vi "generate_double_circ_trajectory.vi"(0 "TrajectoryTS090820Circular2D in":refnum<class "TrajectoryTS090820Circular2D.lvclass">, 1 "trajectory params":T1, 5 "error in (no error)":errorcluster) -> (14 "TrajectoryTS090820Circular2D out":refnum<class "TrajectoryTS090820Circular2D.lvclass">, 15 "trajectory":cluster{dbl[], dbl[], dbl[], dbl[]}, 19 "error out":errorcluster)   [LabVIEW 2010, in "TrajectoryTS090820Circular2D.lvclass"]
uses:
  TrajectoryTS090820Circular2D.lvclass
panel:
  out "dumping amplitude":dbl[](graph)
  out "points BEFORE equal-distribution":cluster{dbl, dbl}[](graph)
  out "intensity":dbl[](array[numeric])
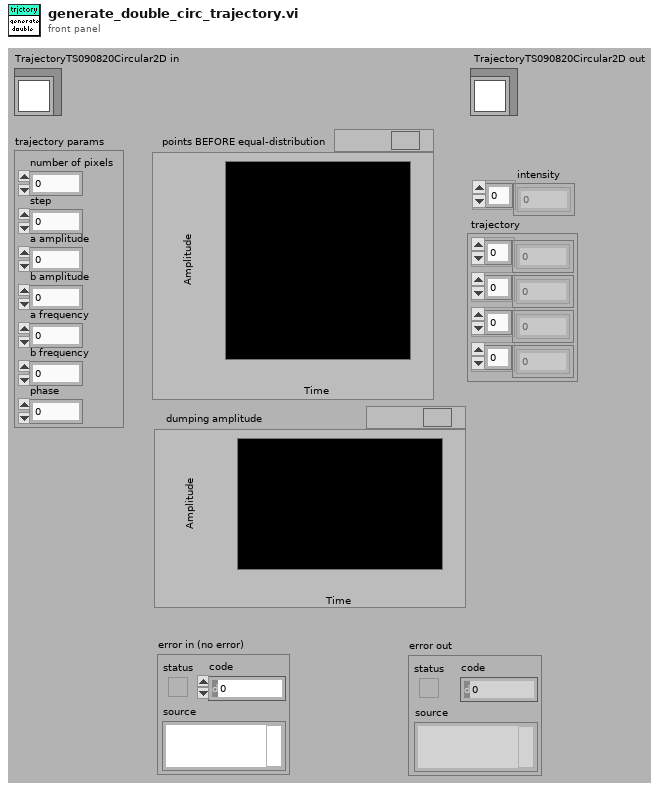
[diagram p1: front panel]
types:
  T1 = cluster{"number of pixels":i32, "step":dbl, "a amplitude":dbl, "b amplitude":dbl, "a frequency":dbl, "b frequency":dbl, "phase":dbl}
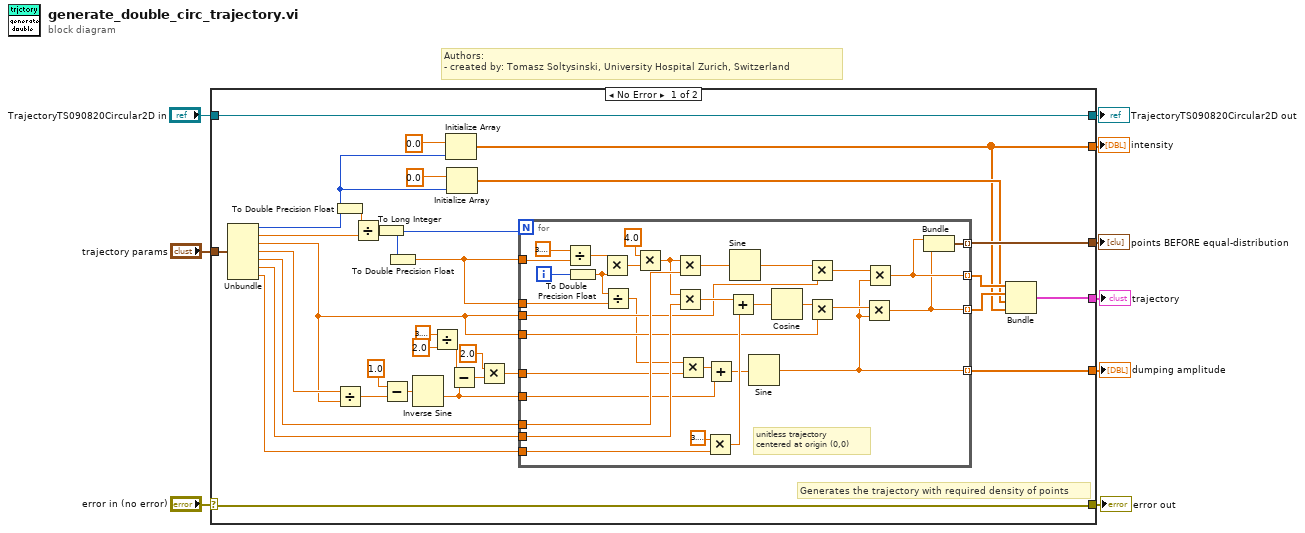
[diagram p0: block diagram]
diagram:
  # "Authors: \n- created by: Tomasz Soltysinski, University Hospital Zurich, Switzerland"
  n1 = case shown="No Error" "error in (no error)" {
    selector: "error in (no error)" -> [w42 w76]
    tunnel: [w42 w76] -> w9
    tunnel: [w24 w75] -> w7
    tunnel: "TrajectoryTS090820Circular2D in" -> [w24 w75]
    tunnel: [w27 _] -> w6
    tunnel: "trajectory params" -> [w37 _]
    tunnel: [w31 _] -> w4
    tunnel: [w26 _] -> w3
    tunnel: [w11 _] -> w1
    frame No Error {
      # "Generates the trajectory with required density of points"
      n2 = Unbundle(w37) -> ("number of pixels"=w36:i32, "step"=w35:dbl, "a amplitude"=w12:dbl, "b amplitude"=w13:dbl, "a frequency"=w34:dbl, "b frequency"=w33:dbl, "phase"=w32:dbl)
      n3 = To Double Precision Float(number=w36) -> (double precision float=w39:dbl)
      n4 = Divide(x=w13, y=w12) -> (x/y=w14:dbl)
      n5 = Divide(x=w39, y=w35) -> (x/y=w38:dbl)
      n6 = To Long Integer(number=w38) -> (32bit integer=w25:i32)
      n7 = Subtract(x=1.0, y=w14) -> (x-y=w22:dbl)
      n8 = To Double Precision Float(number=w25) -> (double precision float=w10:dbl)
      n9 = Inverse Sine(1:w22) -> (0:w15:dbl)
      n10 = Divide(x=3.141592653589793, y=2.0) -> (x/y=w19:dbl)
      n11 = Initialize Array(0.0 ("dimension size"), w36) -> (w27:dbl[])
      n12 = Initialize Array(0.0 ("dimension size"), w36) -> (w28:dbl[])
      n13 = Subtract(x=w19, y=w15) -> (x-y=w18:dbl)
      n14 = Multiply(x=2.0, y=w18) -> (x*y=w16:dbl)
      n15 = for {
        N: w25 -> [_]
        tunnel: w32 -> [w68]
        tunnel: w10 -> [w71]
        tunnel: w34 -> [w67]
        tunnel: w33 -> [w66]
        tunnel: [w49] -> w30 mode=indexing
        tunnel: [w47] -> w29 mode=indexing
        tunnel: [w63] -> w31 mode=indexing
        tunnel: w12 -> [w59]
        tunnel: w12 -> [w58]
        tunnel: w16 -> [w57]
        tunnel: w15 -> [w55]
        tunnel: [w46] -> w11 mode=indexing
        tunnel: w10 -> [w45]
        i -> [w60]
        # "unitless trajectory\ncentered at origin (0,0)"
        n16 = Divide(x=3.141592653589793, y=w71) -> (x/y=w74:dbl)
        n17 = To Double Precision Float(number=w60) -> (double precision float=w44:dbl)
        n18 = Multiply(x=w74, y=w44) -> (x*y=w53:dbl)
        n19 = Divide(x=w44, y=w45) -> (x/y=w43:dbl)
        n20 = Multiply(x=4.0, y=w53) -> (x*y=w52:dbl)
        n21 = Multiply(x=w52, y=w67) -> (x*y=w62:dbl)
        n22 = Multiply(x=w52, y=w66) -> (x*y=w65:dbl)
        n23 = Multiply(x=w43, y=w57) -> (x*y=w56:dbl)
        n24 = Multiply(x=3.141592653589793, y=w68) -> (x*y=w70:dbl)
        n25 = Add(x=w56, y=w55) -> (x+y=w51:dbl)
        n26 = Add(x=w65, y=w70) -> (x+y=w61:dbl)
        n27 = Sine(x=w62) -> (sin(x)=w64:dbl)
        n28 = Sine(x=w51) -> (sin(x)=w46:dbl)
        n29 = Cosine(x=w61) -> (cos(x)=w72:dbl)
        n30 = Multiply(x=w64, y=w59) -> (x*y=w50:dbl)
        n31 = Multiply(x=w72, y=w58) -> (x*y=w48:dbl)
        n32 = Multiply(x=w48, y=w46) -> (x*y=w47:dbl)
        n33 = Multiply(x=w50, y=w46) -> (x*y=w49:dbl)
        n34 = Bundle(w49, w47) -> (w63:cluster{dbl, dbl})  [unwired: 1 in]
      }
      n35 = Bundle(w30, w29, w28, w27) -> (w26:cluster{dbl[], dbl[], dbl[], dbl[]})  [unwired: 1 in]
    }
    frame Error {
    }
  }
  "error out" <- w9
  "TrajectoryTS090820Circular2D out" <- w7
  "intensity" <- w6
  "points BEFORE equal-distribution" <- w4
  "trajectory" <- w3
  "dumping amplitude" <- w1
